vi "Write Module Object.vi"(8 "error in":errorcluster, 10 "cRIO Module Info":T1 {"Product ID" format="%.0x"}) -> (0 "error out":errorcluster, 3 "Module Detection out":refnum<class "Module Detection.lvclass">)   [LabVIEW 2015, in "SMI.lvlib" / "Module Detection.lvclass"]
uses:
  Module Detection.lvclass
  Distributed Devices/Device.lvclass
  Distributed Devices/Controls/DeviceInformation.ctl
panel:
  in  "Module Detection in":refnum<class "Module Detection.lvclass">
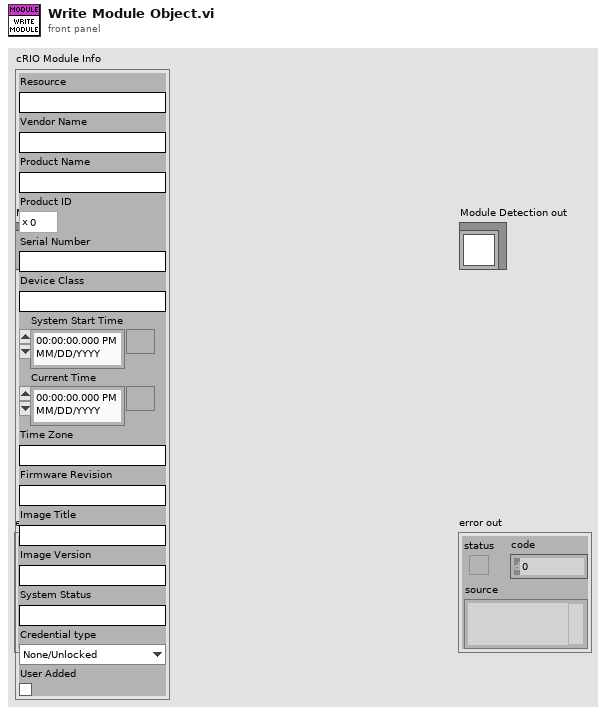
[diagram p1: front panel]
types:
  T1 = typedef "SMI.lvlib/Device.lvclass/DeviceInformation.ctl" = cluster{"Resource":string, "Vendor Name":string, "Product Name":string, "Product ID":u32, "Serial Number":string, "Device Class":string, "System Start Time":timestamp, "Current Time":timestamp, "Time Zone":string, "Firmware Revision":string, "Image Title":string, "Image Version":string, "System Status":string, "Credential type":enum16{"None/Unlocked", "FTP Password", "NIAuth Credentials"}, "User Added":bool}
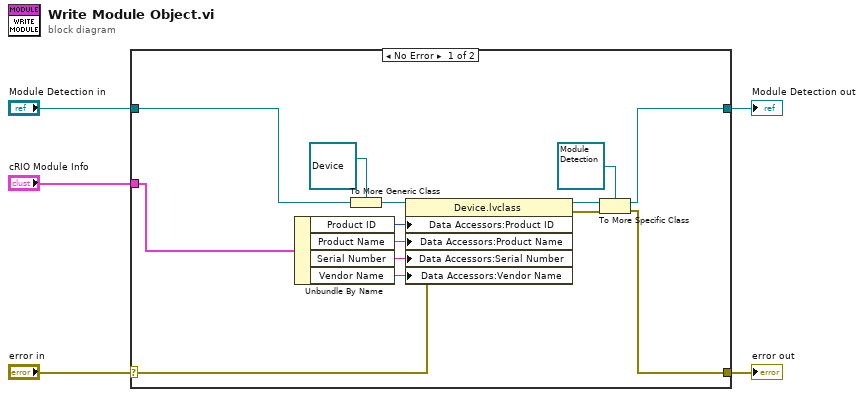
[diagram p0: block diagram]
diagram:
  n1 = case shown="No Error" "error in" {
    selector: "error in" -> [w12 w21]
    tunnel: [w9 w21] -> w4
    tunnel: [w6 w20] -> w2
    tunnel: "Module Detection in" -> [w7 w20]
    tunnel: "cRIO Module Info" -> [w17 _]
    frame No Error {
      n2 = Unbundle By Name(w17) -> ("Product ID"=w16:u32, "Product Name"=w15:string, "Serial Number"=w14:string, "Vendor Name"=w13:string)
      n3 = To More Generic Class(target class=refnum<class "Device.lvclass"> refnum ("RT Management.lvlib:Device.lvclass"), reference=w7) -> (generic class reference=w19:refnum<class "Device.lvclass">)
      n4 = property class="Device.lvclass"(reference=w19, error in=w12, "Data Accessors:Product ID"=w16, "Data Accessors:Product Name"=w15, "Data Accessors:Serial Number"=w14, "Data Accessors:Vendor Name"=w13) -> (reference out=w8:refnum<class "Device.lvclass">, error out=w10:errorcluster)
      n5 = To More Specific Class(target class=refnum<class "Module Detection.lvclass"> refnum ("RT Management.lvlib:Module Detection.lvclass"), reference=w8, error in=w10) -> (specific class reference=w6:refnum<class "Module Detection.lvclass">, error out=w9:errorcluster)
    }
    frame Error {
    }
  }
  "error out" <- w4
  "Module Detection out" <- w2
